vi "Transfer Images Data to UI.vi"(0 "fpga interface in":refnum<k20>, 1 "'stop' notifier":refnum<notifier>, 2 "queue out":refnum<queue>, 3 "measure call context in":refnum<class "Measure Call Context.lvclass">, 5 "Active Channel":string[](array[string]), 7 "display channel number":i32, 11 "error in":errorcluster, 12 "References":T1, 13 "raw display notifier":refnum<notifier>) -> (4 "fpga interface out":refnum<k20>, 15 "error out":errorcluster)   [LabVIEW 2025, in "Automotive Vision.lvclass"]
doc: "Handles frame grabbing, and prepare data for sendig it to the UI."
uses:
  Automotive Vision.lvclass
  <vilib>/Plug-In SDKs/Measurements/Measure Call Context/Measure Call Context.lvclass
  <vilib>/rvi/interface/nirviReadWriteControl/nirviReadWriteControl.xnode
  Automotive Vision.lvclass/Automotive Vision.ctl
  deps/NI148X/Getting Started/Host/Common/GettingStarted_Common_148X_Host.lvlib
  deps/NI148X/Getting Started/Host/Common/Types/148x_Common_FPGA_Reference.ctl
  <instrlib>/FlexRIO/CSI-2/v2/Common/Types/LLP Data Type.ctl
  <instrlib>/FlexRIO/CSI-2/v2/Common/NI CSI-2 API Common v2.lvlib
  Automotive-Vision OOB Data Transfer/Automotive-Vision OOB Data Transfer.lvlib
  Measurement Results.ctl
  NiFpgaLv.dll
  <vilib>/Utility/error.llb/Error Cluster From Error Code.vi
  <vilib>/rvi/interface/Simulation/niFpgaSimulationCallBeginRW.vi
  <vilib>/rvi/errors/niLvFpgaAdjustHostInterfaceError.vi
  <vilib>/vision/Image Controls.llb/IMAQ Image.ctl
  deps/NI148X/Getting Started/Host/Common/Types/RAW Interpretation for Display.ctl
  deps/NI148X/Getting Started/Host/Common/Types/Serial Channel Display Parameters.ctl
panel:
  out "Image Pixels (U32)":u32[](array[numeric])
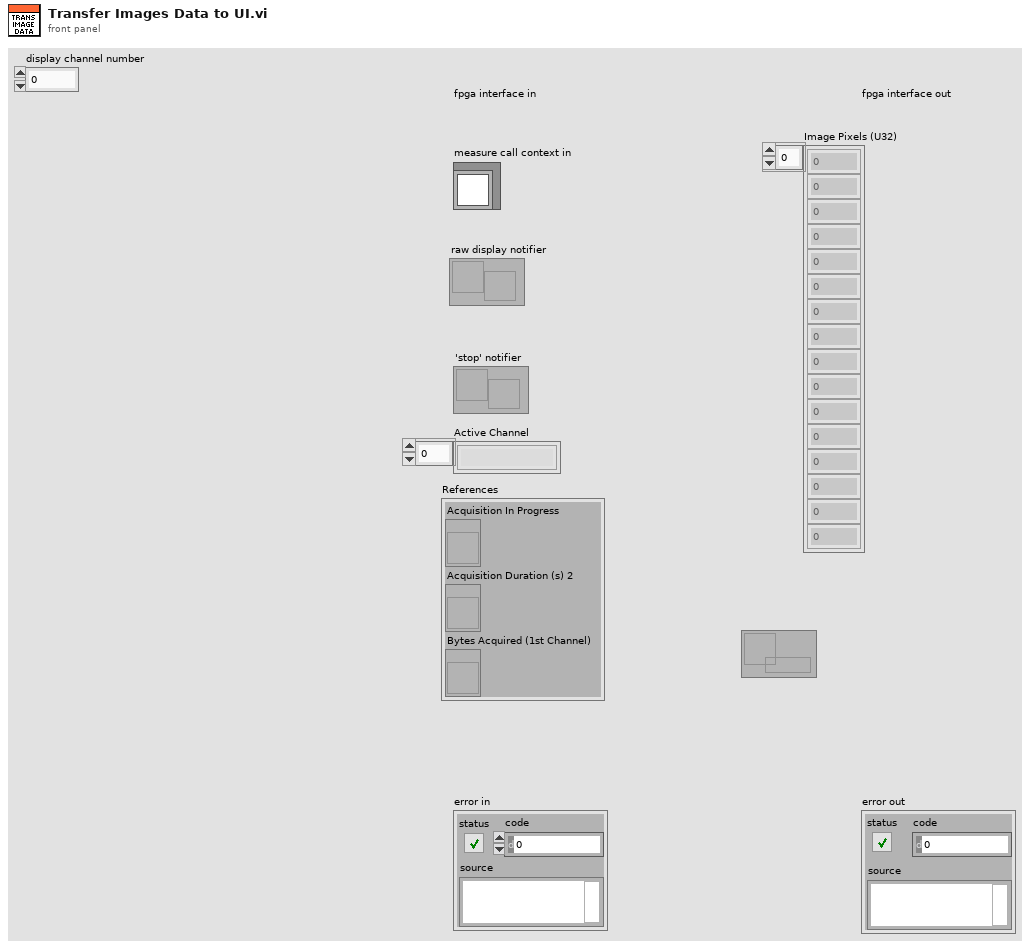
[diagram p1: front panel]
types:
  T1 = cluster{"Acquisition In Progress":refnum<vi>, "Acquisition Duration (s) 2":refnum<vi>, "Bytes Acquired (1st Channel)":refnum<vi>}
  T2 = typedef "NI CSI-2 API Common v2.lvlib/LLP Data Type.ctl" = enum8{"Frame Start", "Frame End", "Line Start", "Line End", "End of Transmission", "Reserved 0", "Reserved 1", "Reserved 2", "Generic Short Packet 1", "Generic Short Packet 2", "Generic Short Packet 3", "Generic Short Packet 4", "Generic Short Packet 5", "Generic Short Packet 6", "Generic Short Packet 7", "Generic Short Packet 8", "Null", "Blanking Data", "Embedded 8-bit non Image Data", "Generic Long Packet 1", "Generic Long Packet 2", "Generic Long Packet 3", "Generic Long Packet 4", "Reserved 3", "YUV420 8-bit", "YUV420 10-bit", "Legacy YUV420 8-bit", "Reserved 4", "YUV420 8-bit Chroma Shifted", "YUV420 10-bit Chroma Shifted", "YUV422 8-bit", "YUV422 10-bit", "RGB444", "RGB555", "RGB565", "RGB666", "RGB888", "Reserved 5", "Reserved 6", "RAW 24", "RAW 6", "RAW 7", "RAW 8", "RAW 10", "RAW 12", "RAW 14", "RAW 16", "RAW 20", "User Defined 8-bit Data 1", "User Defined 8-bit Data 2", "User Defined 8-bit Data 3", "User Defined 8-bit Data 4", "User Defined 8-bit Data 5", "User Defined 8-bit Data 6", "User Defined 8-bit Data 7", "User Defined 8-bit Data 8", "USL Command", "Reserved 7", "Reserved 8", "Reserved 9", "Reserved 10", "Reserved 11", "Reserved 12", "LRTE EPD Spacer"}
  T3 = cluster{"serial channel":fxp<+,3,3>, "frame number":u16, "data type":T2, "width":u16, "height":u16, "image bytes":u32, "total bytes":u32, "little endian":bool, "Status":string}
  T4 = typedef "GettingStarted_Common_148X_Host.lvlib/148x_Common_FPGA_Reference.ctl" = refnum<k20>
  T5 = cluster{"Status Data":cluster{"serial channel":fxp<+,3,3>, "frame number":u16, "data type":T2, "width":u16, "height":u16, "image bytes":u32, "total bytes":u32, "little endian":bool, "Status":string}, "Image Pixels (U32)":u32[], "FrameCount":u64, "SOURCE RATE (fps)":dbl}
  T6 = typedef "GettingStarted_Common_148X_Host.lvlib/Serial Channel Display Parameters.ctl" = cluster{"images":cluster{"grayscale":T7, "color":T7}, "RAW parameters":cluster{"interpretation":T8, "bayer parameters":cluster{"pattern":i32, "algorithm":i32, "red gain":dbl, "green gain":dbl, "blue gain":dbl}}}
  T7 = typedef "IMAQ Image.ctl" = refnum<image>
  T8 = typedef "GettingStarted_Common_148X_Host.lvlib/RAW Interpretation for Display.ctl" = enum16{"Grayscale", "Bayer", "RGB", "YUV422", "YUV420", "Legacy YUV420"}
  T9 = typedef "GettingStarted_Common_148X_FPGA.lvlib/Image Metadata.ctl" = cluster{"serial channel":fxp<+,3,3>, "frame number":u16, "data type":T2, "width":u16, "height":u16, "image bytes":u32, "total bytes":u32, "little endian":bool}
  T10 = typedef "Automotive-Vision OOB Data Transfer.lvlib/OOB to Logic Data.ctl" = cluster{"PauseResume":bool, "ExportPath":string, "ExportType":u16, "Export":bool}
  T11 = typedef "Automotive Vision.lvclass/Measurement Results.ctl" = cluster{"ACQ. IN PROGRESS":bool, "IMAGE PIXEL DATA":u32[], "ACQ. DURATION (s)":dbl, "SOURCE RATE (fps)":dbl, "BYTES ACQUIRED":u64, "FRAME COUNT":u64, "POC VOLTAGE (V)":dbl, "POC CURRENT (A)":dbl, "ERROR":bool, "STATE MESSAGE":string, "IMAGE DATA":string, "OOB gRPC Port":i32, "HEIGHT":u64, "WIDTH":u64, "IMAGE SIZE":u64}
  T12 = cluster{"image pixel data fifo overflow":bool, "image metadata fifo overflow":bool}[]
  T13 = cluster{"image pixel data fifo overflow":bool, "image metadata fifo overflow":bool}
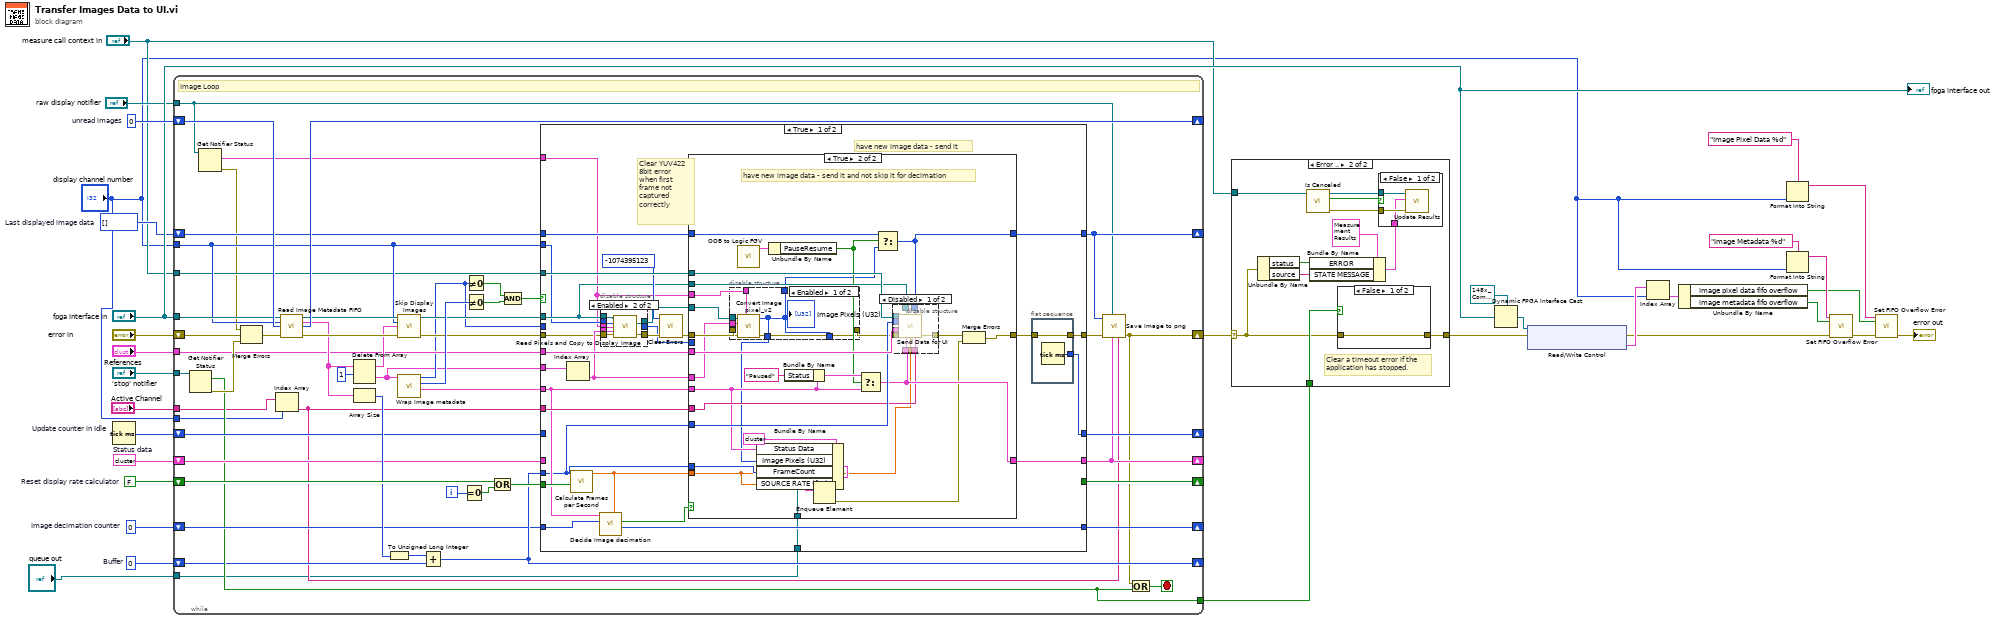
[diagram p0: block diagram]
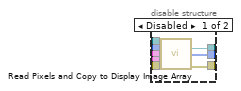
[diagram p2: hidden frame]
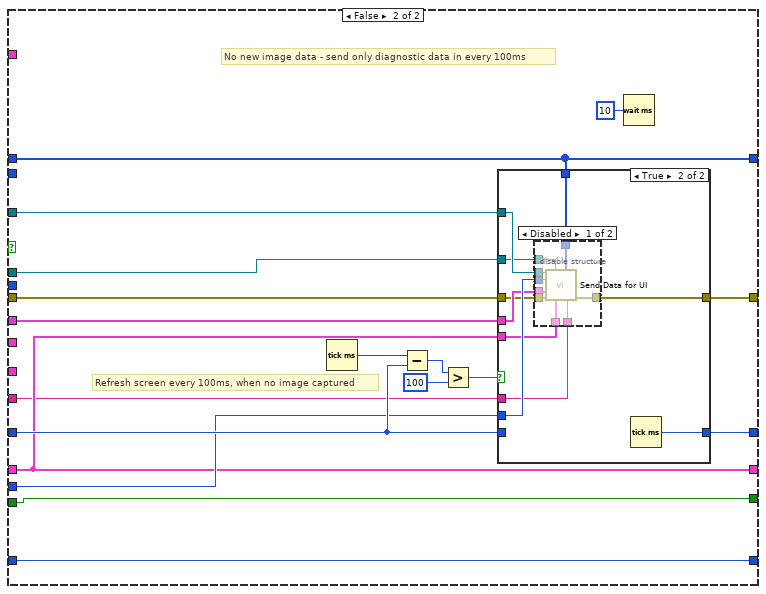
[diagram p6: hidden frame]
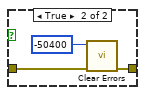
[diagram p11: hidden frame]
diagram:
  w6 = T3 {"serial channel"=0.0, "frame number"=0, "data type"=enum."Frame Start", "width"=0, "height"=0, "image bytes"=0, "total bytes"=0, "little endian"=FALSE, "Status"="Ready for Acquisition"}  # Status data
  w9 = u32 0  # Image decimation counter
  w10 = u32[] []  # Last displayed image data
  w16 = u32 0  # Buffer
  w17 = FALSE  # Reset display rate calculator
  w32 = u32 0  # unread images
  n1 = Tick Count (ms) "Update counter in Idle"() -> (millisecond timer value=w11:u32)
  n2 = while {
    shift-right: [w41] -> w15
    shift-left: "error in" -> [w59]
    tunnel: "fpga interface in" -> [w62]
    shift-right: [w82] -> _
    shift-left: w32 -> [w73]
    tunnel: "display channel number" -> [w58]
    shift-right: [w77] -> _
    shift-left: w17 -> [w74]
    shift-right: [w64] -> _
    shift-left: w16 -> [w45]
    tunnel: [w47] -> w13
    tunnel: "'stop' notifier" -> [w61]
    shift-right: [w56] -> _
    shift-left: w11 -> [w57]
    shift-right: [w44] -> _
    shift-left: w10 -> [w55]
    shift-right: [w53] -> _
    shift-left: w9 -> [w54]
    tunnel: "References" -> [w52]
    tunnel: "measure call context in" -> [w51]
    shift-right: [w42] -> _
    shift-left: w6 -> [w50]
    tunnel: "raw display notifier" -> [w38]
    tunnel: "Active Channel" -> [w40]
    tunnel: "display channel number" -> [w34]
    tunnel: "queue out" -> [w33]
    i -> [w81]
    stop <- w83 stop-if-true
    # "Image Loop"
    n3 = Get Notifier Status(notifier=w61) -> (current notification=w47:bool, error out=w84:errorcluster)  [unwired: 1 in, 3 out]
    n4 = Get Notifier Status(notifier=w38) -> (current notification=w36:T6[], error out=w37:errorcluster)  [unwired: 1 in, 3 out]
    n5 = Merge Errors(w37, w59, w84) -> (w60:errorcluster)
    n6 = Index Array(array=w40, index=w34) -> (element=w39:string)
    n7 = call "Read Image Metadata FIFO.vi"("fpga inteface in"=w62, "display channel number"=w58, "number of images"=w73, "error in (no error)"=w60) -> ("fpga interface out"=w70:refnum<k20>, "image metadata"=w63:T9[], "images remaining"=w82:u32, "error out"=w67:errorcluster)  [unwired: 8 in]
    n8 = Delete From Array(array=w63, length=1) -> (deleted portion=w35:T9[], array with subset deleted=w66:T9[])  [unwired: 1 in]
    n9 = Array Size(array=w63) -> (size(s)=w65:i32)
    n10 = To Unsigned Long Integer(number=w65) -> (unsigned 32bit integer=w46:u32)
    n11 = call "Skip Display Images.vi"("fpga interface in"=w70, "display channel number"=w58, "image metadata"=w66, "error in (no error)"=w67) -> ("fpga interface out"=w69:refnum<k20>, "error out"=w68:errorcluster)  [unwired: 10 in]
    n12 = call "Wrap Image metadata.vi"("image metadata"=w35) -> ("element"=w49:T3, "Numeric"=w72:i32, "total bytes"=w48:u32)  [unwired: 8 in]
    n13 = Add(x=w46, y=w45) -> (x+y=w64:u32)
    n14 = Equal To 0?(x=w81) -> (x = 0?=w75:bool)
    n15 = Not Equal To 0?(x=w48) -> (x != 0?=w79:bool)
    n16 = Not Equal To 0?(x=w72) -> (x != 0?=w80:bool)
    n17 = Compound Arithmetic op=OR(w74, w75) -> (w76:bool)
    n18 = Compound Arithmetic op=AND(w79, w80) -> (w78:bool)
    n19 = case shown="True" w78 {
      tunnel: w68 -> [w88 w180]
      tunnel: w69 -> [w92 w178]
      tunnel: w58 -> [w91 _]
      tunnel: [w110 w187] -> w43
      tunnel: w76 -> [w102 w194]
      tunnel: [_ w194] -> w77
      tunnel: w64 -> [w85 w184]
      tunnel: w48 -> [_ _]
      tunnel: w49 -> [w98 _]
      tunnel: w51 -> [w112 w181]
      tunnel: w52 -> [w111 w195]
      tunnel: w57 -> [_ w186]
      tunnel: [w109 w188] -> w56
      tunnel: w55 -> [w107 w185]
      tunnel: [w108 w185] -> w44
      tunnel: w54 -> [w106 w183]
      tunnel: [w105 w183] -> w53
      tunnel: w50 -> [_ w182]
      tunnel: [w103 w182] -> w42
      tunnel: w39 -> [w101 w179]
      tunnel: w36 -> [w90 _]
      tunnel: w35 -> [w99 _]
      tunnel: w33 -> [w86 _]
      frame True {
        # "Clear YUV422 8bit error when first frame not captured correctly"
        # "have new image data - send it"
        n20 = Index Array(array=w99) -> (element=w89:T9)  [unwired: 1 in]
        n21 = call <vilib>:"Calculate Frames per Second.vi"("Reset"=w102, "Buffer Number"=w85) -> ("Acquired Frames/s"=w97:dbl)  [unwired: 7 in, 2 out]
        n22 = call "Decide Image decimation.vi"("FPS"=w97, "Image decimation counter in"=w106, "element in"=w98) -> ("Image decimation counter out"=w105:u32, "send current image data"=w104:bool)  [unwired: 7 in]
        n23 = disable-structure shown="Enabled" {
          disable-tunnel: [w120 w126] -> w94
          disable-tunnel: [w119 w125] -> w93
          disable-tunnel: w92 -> [w118 w124]
          disable-tunnel: w91 -> [w117 w123]
          disable-tunnel: w90 -> [w116 w122]
          disable-tunnel: w89 -> [w115 w121]
          disable-tunnel: w88 -> [w114 w126]
          disable-tunnel: [w113 _] -> w87
          frame Disabled {
            n24 = call "Read Pixels and Copy to Display Image Array.vi"("fpga interface in"=w118, "display channel number"=w117, "serial channel display parameters"=w116, "image metadata"=w115, "error in (no error)"=w114) -> ("display image"=w119:T7, "Pixel Data"=w113:u32[], "error out"=w120:errorcluster)  [unwired: 7 in, 1 out]
          }
          frame Enabled {
            n25 = call "Read Pixels and Copy to Display Image.vi"("fpga interface in"=w124, "display channel number"=w123, "serial channel display parameters"=w122, "image metadata"=w121) -> ("display image"=w125:T7)  [unwired: 9 in, 2 out]
          }
        }
        n26 = call <vilib>:"Clear Errors.vi"("error in (no error)"=w94, "specific error code to clear (0: all)"=-1074395123) -> ("error out"=w95:errorcluster)  [unwired: 4 in, 1 out]
        n27 = case shown="True" w104 {
          tunnel: [w127 w137] -> w100
          tunnel: w97 -> [_ w130]
          tunnel: w98 -> [w128 w134]
          tunnel: w112 -> [_ w157]
          tunnel: w111 -> [_ w156]
          tunnel: [w129 w155] -> w108
          tunnel: w85 -> [_ w154]
          tunnel: w107 -> [w129 w153]
          tunnel: [w128 w152] -> w103
          tunnel: w92 -> [_ w151]
          tunnel: w101 -> [_ w145]
          tunnel: w95 -> [w127 w144]
          tunnel: w93 -> [_ w142]
          tunnel: w89 -> [_ w141]
          tunnel: w90 -> [_ w140]
          tunnel: w87 -> [_ _]
          tunnel: w86 -> [_ w138]
          tunnel: w85 -> [_ w131]
          frame False {
            # "have new image data - but skip the sending to not overload UI with data transfer"
          }
          frame True {
            # "have new image data - send it and not skip it for decimation"
            n28 = disable-structure shown="Enabled" {
              disable-tunnel: w144 -> [w174 w175]
              disable-tunnel: [w173 w175] -> w143
              disable-tunnel: w142 -> [w172 _]
              disable-tunnel: w141 -> [w171 _]
              disable-tunnel: w140 -> [w170 _]
              disable-tunnel: [w169 _] -> w139
              disable-tunnel: [w169 _] -> _
              disable-tunnel: [w169 _] -> w133
              frame Enabled {
                n29 = call "Convert Image pixel_v2.vi"("serial channel display parameters"=w170, "error in"=w174, "image metadata"=w171, "Refnum in"=w172) -> ("error out"=w173:errorcluster, "Image Pixels (U32)"=w169:u32[])  [unwired: 6 in]
                "Image Pixels (U32)" <- w169
              }
              frame Disabled {
              }
            }
            n30 = call "OOB to Logic FGV.vi"() -> ("OOB to Logic Data out"=w147:T10)  [unwired: 10 in, 1 out]
            n31 = Bundle By Name(cluster=T5 {"Status Data"={"serial channel"=0.0, "frame number"=0, "data type"=enum."Frame Start", "width"=0, "height"=0, "image bytes"=0, "total bytes"=0, "little endian"=FALSE, "Status"=""}, "Image Pixels (U32)"=[], "FrameCount"=0, "SOURCE RATE (fps)"=0.0}, "Status Data"=w134, "Image Pixels (U32)"=w133, "FrameCount"=w131, "SOURCE RATE (fps)"=w130) -> (w132:T5)
            n32 = Unbundle By Name(w147) -> ("PauseResume"=w146:bool)
            n33 = Bundle By Name(cluster=w134, "Status"="Paused") -> (w149:T3)
            n34 = Enqueue Element(queue=w138, element=w132) -> (error out=w136:errorcluster)  [unwired: 2 in, 2 out]
            n35 = Select(t=w149, s=w146, f=w134) -> (s? t:f=w152:T3)
            n36 = Select(t=w153, s=w146, f=w139) -> (s? t:f=w155:u32[])
            n37 = disable-structure shown="Disabled" {
              disable-tunnel: w130 -> [w167 _]
              disable-tunnel: w157 -> [w166 _]
              disable-tunnel: w156 -> [w165 _]
              disable-tunnel: w155 -> [w164 _]
              disable-tunnel: w154 -> [w163 _]
              disable-tunnel: w152 -> [w162 _]
              disable-tunnel: w151 -> [w161 _]
              disable-tunnel: [w160 w168] -> w150
              disable-tunnel: w145 -> [w159 _]
              disable-tunnel: w143 -> [w158 w168]
              frame Disabled {
                n38 = call "Send Data for UI.vi"("Measure Call Context in"=w166, "fpga interface in"=w161, "Last displayed image data"=w164, "FrameCount"=w163, "References"=w165, "error in"=w158, "Status data"=w162, "SOURCE RATE (fps)"=w167, "Active Channel"=w159) -> ("error out"=w160:errorcluster)  [unwired: 6 in]
              }
              frame Enabled {
              }
            }
            n39 = Merge Errors(w150, w136) -> (w137:errorcluster)
          }
        }
        n40 = flat-sequence {
          tunnel: [w177] -> w110
          tunnel: w100 -> [w177]
          tunnel: [w176] -> w109
          frame #0 {
            n41 = Tick Count (ms)() -> (millisecond timer value=w176:u32)
          }
        }
      }
      frame False {
        # "Refresh screen every 100ms, when no image captured"
        # "No new image data - send only diagnostic data in every 100ms"
        n42 = Tick Count (ms)() -> (millisecond timer value=w192:u32)
        n43 = Subtract(x=w192, y=w186) -> (x-y=w191:u32)
        n44 = Greater?(x=w191, y=u32 100) -> (0:w189:bool)
        n45 = case shown="True" w189 {
          tunnel: w180 -> [w197 w200]
          tunnel: [w197 w207] -> w187
          tunnel: w182 -> [_ w202]
          tunnel: w195 -> [_ w203]
          tunnel: [w196 w206] -> w188
          tunnel: w186 -> [w196 _]
          tunnel: w185 -> [_ w205]
          tunnel: w184 -> [_ w204]
          tunnel: w181 -> [_ w201]
          tunnel: w179 -> [_ w199]
          tunnel: w178 -> [_ w198]
          frame False {
          }
          frame True {
            n46 = disable-structure shown="Disabled" {
              disable-tunnel: [w216 w217] -> w207
              disable-tunnel: w205 -> [w215 _]
              disable-tunnel: w204 -> [w214 _]
              disable-tunnel: w203 -> [w213 _]
              disable-tunnel: w202 -> [w212 _]
              disable-tunnel: w201 -> [w211 _]
              disable-tunnel: w200 -> [w210 w217]
              disable-tunnel: w199 -> [w209 _]
              disable-tunnel: w198 -> [w208 _]
              frame Disabled {
                n47 = call "Send Data for UI.vi"("Measure Call Context in"=w211, "fpga interface in"=w208, "Last displayed image data"=w215, "FrameCount"=w214, "References"=w213, "error in"=w210, "Status data"=w212, "Active Channel"=w209) -> ("error out"=w216:errorcluster)  [unwired: 7 in]
              }
              frame Enabled {
              }
            }
            n48 = Tick Count (ms)() -> (millisecond timer value=w206:u32)
          }
        }
        n49 = Wait (ms)(milliseconds to wait=u32 10) -> ()  [unwired: 1 out]
      }
    }
    n50 = call "Save Image to png.vi"("Channel"=w39, "image metadata"=w42, "raw display notifier"=w38, "error in"=w43, "Last displayed image data"=w44) -> ("error out"=w41:errorcluster)  [unwired: 6 in]
    n51 = Compound Arithmetic op=OR(w41, w47) -> (w83:bool)
  }
  n52 = case shown="Error .." w15 {
    selector: w15 -> [w218 w222]
    tunnel: [w218 w229] -> w27
    tunnel: w13 -> [_ w228]
    tunnel: "measure call context in" -> [_ w219]
    frame No Error {
    }
    frame Error {
      # "Clear a timeout error if the application has stopped."
      n53 = Unbundle By Name(w222) -> ("status"=w221:bool, "source"=w220:string)
      n54 = call <vilib>:"Is Canceled.vi"("measure call context in"=w219) -> ("error out"=w226:errorcluster, "is canceled?"=w225:bool, "measure call context out"=w227:refnum<class "Measure Call Context.lvclass">)  [unwired: 8 in]
      n55 = Bundle By Name(cluster=T11 {"ACQ. IN PROGRESS"=FALSE, "IMAGE PIXEL DATA"=[], "ACQ. DURATION (s)"=0.0, "SOURCE RATE (fps)"=0.0, "BYTES ACQUIRED"=0, "FRAME COUNT"=0, "POC VOLTAGE (V)"=0.0, "POC CURRENT (A)"=0.0, "ERROR"=FALSE, "STATE MESSAGE"="", "IMAGE DATA"="", "OOB gRPC Port"=0, "HEIGHT"=0, "WIDTH"=0, "IMAGE SIZE"=0} ("Measurement Results"), "ERROR"=w221, "STATE MESSAGE"=w220) -> (w223:T11)
      n56 = case shown="False" w228 {
        tunnel: w222 -> [w233 w236]
        tunnel: [w233 w234] -> w229
        frame False {
        }
        frame True {
          n57 = call <vilib>:"Clear Errors.vi"("error in (no error)"=w236, "specific error code to clear (0: all)"=-50400 ("y")) -> ("error out"=w234:errorcluster)  [unwired: 4 in, 1 out]
        }
      }
      n58 = case shown="False" w225 {
        tunnel: w227 -> [w232 _]
        tunnel: w226 -> [w231 _]
        tunnel: w223 -> [w230 _]
        frame False {
          n59 = call <vilib>:"Update Results.vi"("error in"=w231, "measurement results"=w230, "measure call context in"=w232) -> ()  [unwired: 7 in, 2 out]
        }
        frame True {
        }
      }
    }
  }
  n60 = Dynamic FPGA Interface Cast(Session In=T4 refnum ("FPGA VI Reference Out"), Type="fpga interface in") -> (Session Out=w28:T4)
  n61 = xnode ("Read/Write Control")("FPGA VI Reference In"=w28, "error in"=w27) -> ("error out"=w26:errorcluster, "display channel status"=w30:T12)  [unwired: 1 out]
  n62 = Index Array(array=w30, index="display channel number") -> (element=w31:T13)
  n63 = Unbundle By Name(w31) -> ("image pixel data fifo overflow"=w19:bool, "image metadata fifo overflow"=w18:bool)
  n64 = Format Into String(format string="Image Pixel Data %d", "display channel number") -> (resulting string=w21:string)  [unwired: 2 in, 1 out]
  n65 = Format Into String(format string="Image Metadata %d", "display channel number") -> (resulting string=w20:string)  [unwired: 2 in, 1 out]
  n66 = call "Set FIFO Overflow Error.vi"("fifo name"=w20, "overflow"=w18, "error in (no error)"=w26) -> ("error out"=w23:errorcluster)  [unwired: 12 in]
  n67 = call "Set FIFO Overflow Error.vi"("fifo name"=w21, "overflow"=w19, "error in (no error)"=w23) -> ("error out"=→"error out":errorcluster)  [unwired: 12 in]
  "fpga interface out" <- "fpga interface in"
